vi "ExampleQueryServer.vi"() -> ()   [LabVIEW 2019]
uses:
  VIs/labview-grpc-query-server.lvlib
  VIs/gprc-support.lvlib
panel:
  in  "Server Key File (.key)":path
  in  "Server Certificate File (.crt)":path
  in  "stop":bool
  in  "Server Address":string="0.0.0.0:50051"
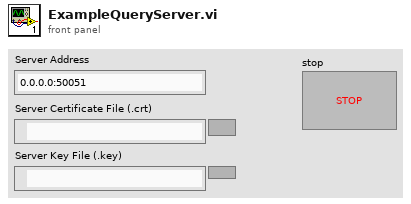
[diagram p1: front panel]
types:
  T1 = typedef "gprc-support.lvlib/grpcId.ctl" = u64
  T2 = cluster{"QueryServer_Invoke":refnum<user-event>, "QueryServer_Query":refnum<user-event>, "QueryServer_Register":refnum<user-event>, "QueryServer_TestDataTypes":refnum<user-event>, "serverId":T1}
  T3 = typedef "labview-grpc-query-server.lvlib/QueryServer_gRPCid.ctl" = u64
  T4 = typedef "labview-grpc-query-server.lvlib/QueryServer_TestDataTypesParameters.ctl" = cluster{"Root":string, "Repeated String":string[], "Repeated Int32":i32[], "Root Int32":i32, "Root Bool":bool, "Repeated Double":dbl[], "Root Double":dbl, "Repeated Bool":bool[], "Root Float":sgl, "Repeated Float":sgl[], "DataTypeTest":T5, "Repeated Nested":T5[]}
  T5 = typedef "labview-grpc-query-server.lvlib/QueryServer_DataTypeTest.ctl" = cluster{"Bool Value":bool, "Int Value":i32, "Float Value":sgl, "Double Value":dbl}
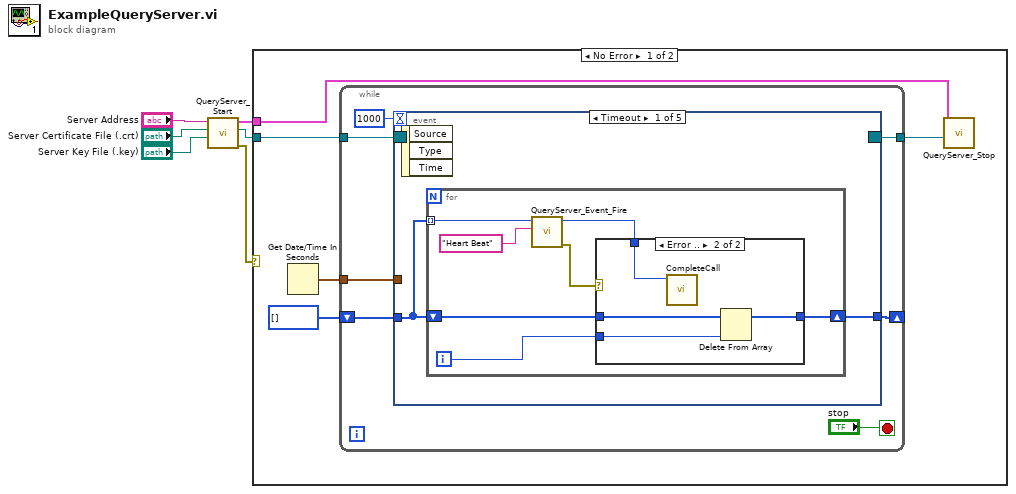
[diagram p0: block diagram]
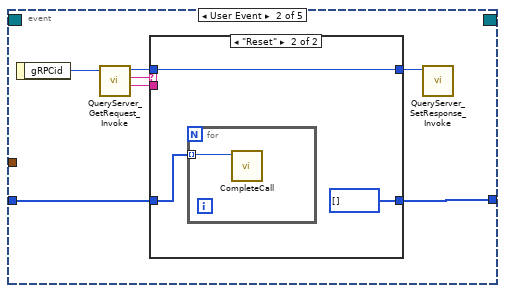
[diagram p3: hidden frame]
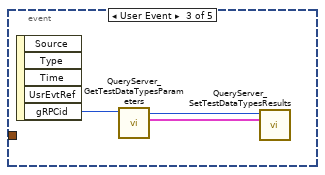
[diagram p5: hidden frame]
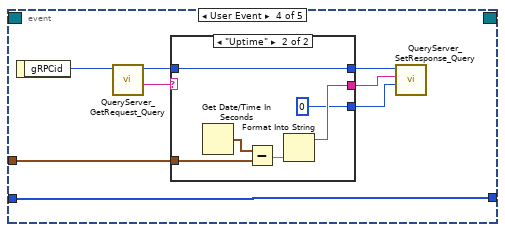
[diagram p6: hidden frame]
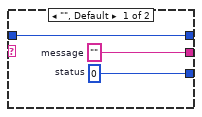
[diagram p7: hidden frame]
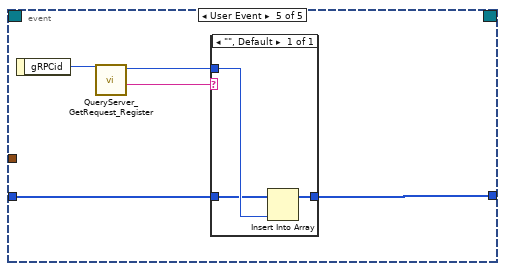
[diagram p8: hidden frame]
diagram:
  n1 = call "QueryServer_Start.vi"("Server Key File (.key)"="Server Key File (.key)", "Server Certificate File (.crt)"="Server Certificate File (.crt)", "Server Address"="Server Address") -> ("error out"=w2:errorcluster, "Event Registration Refnum"=w1:refnum<event-registration>, "Server Info"=w5:T2)  [unwired: 5 in]
  n2 = case shown="No Error" w2 {
    tunnel: w5 -> [w9 _]
    tunnel: w1 -> [w7 _]
    frame No Error {
      n3 = Get Date/Time In Seconds() -> (seconds since 1Jan1904=w11:timestamp)
      n4 = while {
        tunnel: [w17] -> w8
        tunnel: w11 -> [w16]
        shift-right: [w14] -> _
        shift-left: u64[] [] -> [w13]
        tunnel: w7 -> [w12]
        stop <- "stop" stop-if-true
        n5 = event shown="[0] Timeout" {
          selector: w12 -> [_ _ _ _ _]
          dyn-events: [_ _ _ _ _] -> w17
          timeout: 1000 -> [_ _ _ _ _]
          tunnel: w16 -> [_ _ _ w51 _]
          tunnel: [w19 w33 _ w50 w68] -> w14
          tunnel: w13 -> [w20 w34 _ w50 w67]
          event Timeout {
            n6 = event-data() -> ()  [unwired: 1 in, 3 out]
            n7 = for {
              tunnel: w20 -> [w27] mode=indexing
              shift-right: [w23] -> w19
              shift-left: w20 -> [w22]
              i -> [w24]
              n8 = call "QueryServer_Event_Fire.vi"("eventdata"="Heart Beat", "gRPCid"=w27) -> ("error out"=w25:errorcluster, "gRPCid out"=w21:T1)  [unwired: 8 in]
              n9 = case shown="Error .." w25 {
                tunnel: w22 -> [w28 w32]
                tunnel: w24 -> [_ w31]
                tunnel: [w28 w30] -> w23
                tunnel: w21 -> [_ w29]
                frame No Error {
                }
                frame Error {
                  n10 = call "CompleteCall.vi"("gRPCid"=w29) -> ()  [unwired: 9 in, 1 out]
                  n11 = Delete From Array(array=w32, index=w31) -> (array with subset deleted=w30:u64[])  [unwired: 1 in, 1 out]
                }
              }
            }
          }
          event User Event {
            n12 = event-data() -> ("gRPCid"=w39:T3)  [unwired: 1 in]
            n13 = call "QueryServer_GetRequest_Invoke.vi"("gRPCid"=w39) -> ("parameter"=w35:string, "command"=w38:string, "gRPCid out"=w37:T1)  [unwired: 5 in, 1 out]
            n14 = case shown="\"Reset\"" w38 {
              tunnel: w37 -> [w41 w42]
              tunnel: [w41 w42] -> w36
              tunnel: w35 -> [_ _]
              tunnel: w34 -> [w40 w44]
              tunnel: [w40 u64[] []] -> w33
              frame "", Default {
              }
              frame "Reset" {
                n15 = for {
                  tunnel: w44 -> [w45] mode=indexing
                  n16 = call "CompleteCall.vi"("gRPCid"=w45) -> ()  [unwired: 9 in, 1 out]
                }
              }
            }
            n17 = call "QueryServer_SetResponse_Invoke.vi"("gRPCid"=w36) -> ()  [unwired: 9 in, 1 out]
          }
          event User Event {
            n18 = event-data() -> ("gRPCid"=w48:T3)  [unwired: 1 in, 4 out]
            n19 = call "QueryServer_GetTestDataTypesParameters.vi"("gRPCid"=w48) -> ("TestDataTypesParameters"=w47:T4, "gRPCid out"=w46:T1)  [unwired: 6 in, 1 out]
            n20 = call "QueryServer_SetTestDataTypesResults.vi"("TestDataTypesParameters"=w47, "gRPCid"=w46) -> ()  [unwired: 6 in, 2 out]
          }
          event User Event {
            n21 = event-data() -> ("gRPCid"=w56:T3)  [unwired: 1 in]
            n22 = call "QueryServer_GetRequest_Query.vi"("gRPCid"=w56) -> ("gRPCid out"=w55:T1, "query"=w49:string)  [unwired: 7 in, 1 out]
            n23 = case shown="\"Uptime\"" w49 {
              tunnel: w55 -> [w59 w61]
              tunnel: [w59 w61] -> w54
              tunnel: [w58 w62] -> w53
              tunnel: [w57 0 ("status")] -> w52
              tunnel: w51 -> [_ w64]
              frame "", Default {
                w57 = 0  # status
                w58 = ""  # message
              }
              frame "Uptime" {
                n24 = Get Date/Time In Seconds() -> (seconds since 1Jan1904=w65:timestamp)
                n25 = Subtract(x=w65, y=w64) -> (x-y=w63:dbl)
                n26 = Format Into String(w63) -> (resulting string=w62:string)  [unwired: 3 in, 1 out]
              }
            }
            n27 = call "QueryServer_SetResponse_Query.vi"("gRPCid"=w54, "message"=w53, "status"=w52) -> ()  [unwired: 7 in, 1 out]
          }
          event User Event {
            n28 = event-data() -> ("gRPCid"=w70:T3)  [unwired: 1 in]
            n29 = call "QueryServer_GetRequest_Register.vi"("gRPCid"=w70) -> ("gRPCid out"=w69:T1, "eventname"=w66:string)  [unwired: 7 in, 1 out]
            n30 = case shown="\"\", Default" w66 {
              tunnel: w69 -> [w73]
              tunnel: [w72] -> w68
              tunnel: w67 -> [w71]
              frame "", Default {
                n31 = Insert Into Array(array=w71, new element=w73) -> (w72:u64[])  [unwired: 1 in]
              }
            }
          }
        }
      }
      n32 = call "QueryServer_Stop.vi"("Server Info"=w9, "Event Registration Refnum"=w8) -> ()  [unwired: 8 in, 1 out]
    }
    frame Error {
    }
  }
